vi "Check Complete.vi"(8 "error in (no error)":errorcluster, 10 "Amphipods":refnum<class "Amphipod.lvclass">[](array[class]), 11 "Amphipod in":refnum<class "Amphipod.lvclass">) -> (0 "error out":errorcluster, 2 "Complete?":bool, 3 "Amphipod out":refnum<class "Amphipod.lvclass">)   [LabVIEW 2019, in "23.lvlib" / "Amphipod.lvclass"]
uses:
  Amphipod.lvclass
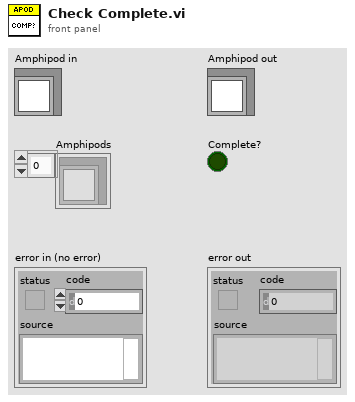
[diagram p1: front panel]
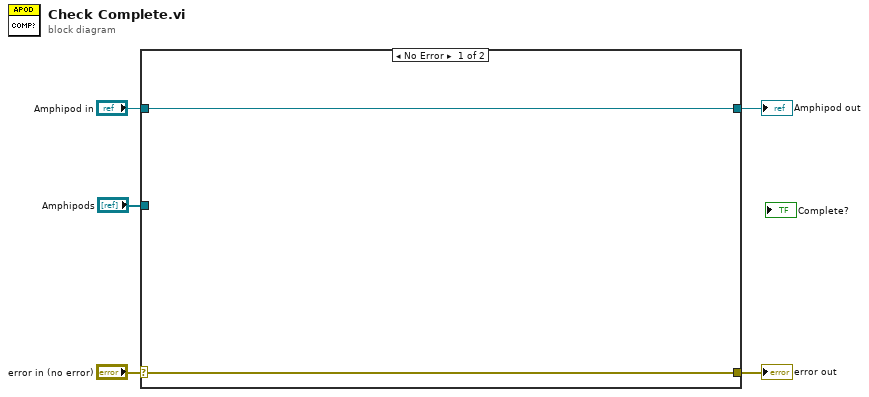
[diagram p0: block diagram]
diagram:
  n1 = case shown="No Error" "error in (no error)" {
    selector: "error in (no error)" -> [w6 w9]
    tunnel: [w6 w9] -> w4
    tunnel: [w7 w8] -> w2
    tunnel: "Amphipod in" -> [w7 w8]
    tunnel: "Amphipods" -> [_ _]
    frame No Error {
    }
    frame Error {
    }
  }
  "error out" <- w4
  "Amphipod out" <- w2
